vi "IO_Level_Sensor.vi"(6 "error IN":errorcluster {"code" format="%x"}) -> (1 "status":bool, 3 "PV (raw)":dbl, 4 "error OUT":errorcluster {"code" format="%x"})   [LabVIEW 2024]
uses:
  <instrlib>/Keyence LK-G3000/Public/clusters/LKIF_FLOATVALUE.ctl
  <instrlib>/Keyence LK-G3000/Public/enums/LKIF_FLOATRESULT.ctl
  <instrlib>/Keyence LK-G3000/Keyence LK-G3000.lvlib
panel:
  out "CalcData2":T1 {"LKIF_FLOATRESULT" items=["VALID", "RANGEOVER_P", "RANGEOVER_N", "WAITING"]}
  out "CalcData1":T1 {"LKIF_FLOATRESULT" items=["VALID", "RANGEOVER_P", "RANGEOVER_N", "WAITING"]}
  out "Trend Graph":cluster{"Value":sgl, "Value":sgl}(graph)
  # "Scaled OUT"
  # "Corrected OUT"
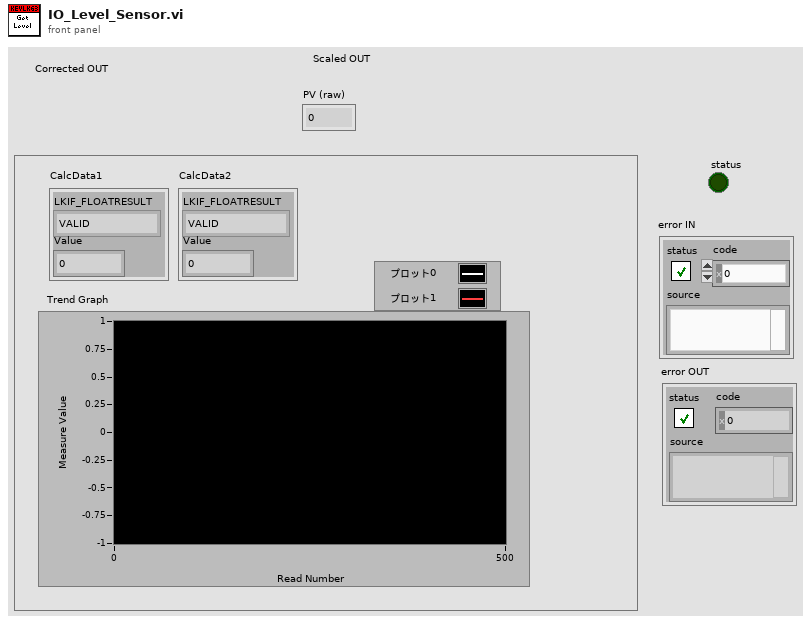
[diagram p1: front panel]
types:
  T1 = typedef "Keyence LK-G3000.lvlib/LKIF_FLOATVALUE.ctl" = cluster{"LKIF_FLOATRESULT":T2, "Value":sgl}
  T2 = typedef "Keyence LK-G3000.lvlib/LKIF_FLOATRESULT.ctl" = i32
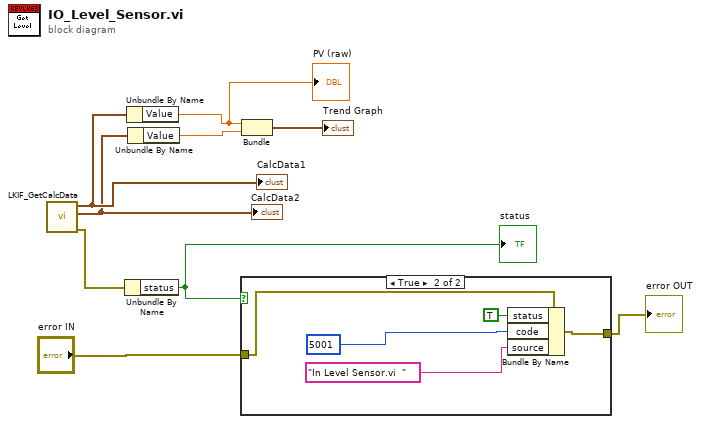
[diagram p0: block diagram]
diagram:
  n1 = call <instrlib>:"LKIF_GetCalcData.vi"() -> ("error out"=w2:errorcluster, "CalcData2"=w8:T1, "CalcData1"=w9:T1)  [unwired: 9 in]
  "CalcData1" <- w9
  "CalcData2" <- w8
  n2 = Unbundle By Name(w2) -> ("status"=w3:bool)
  "status" <- w3
  n3 = Unbundle By Name(w9) -> ("Value"=w1:sgl)
  "PV (raw)" <- w1
  n4 = Unbundle By Name(w8) -> ("Value"=w7:sgl)
  n5 = case shown="True" w3 {
    tunnel: [w10 w14] -> w5
    tunnel: "error IN" -> [w10 w15]
    frame False {
    }
    frame True {
      n6 = Bundle By Name(cluster=w15, "status"=TRUE, "code"=5001 ("[error code] (0)"), "source"="In Level Sensor.vi  " ("[error source] (\" \")")) -> (w14:errorcluster)
    }
  }
  "error OUT" <- w5
  n7 = Bundle("Value"=w1, "Value"=w7) -> (→"Trend Graph":cluster{"Value":sgl, "Value":sgl})  [unwired: 1 in]
